vi "FPGAPowerMeasurement4.vi"() -> ()   [LabVIEW 2009]
uses:
  <vilib>/Waveform/DWDTOps.llb/Digital Pattern Generator (Toggle).vi
  <vilib>/express/express analysis/Spectral/XNode/ExpressSpectralMeasurementsBlockNode.xnode
  <vilib>/express/express analysis/Spectral/Block/exnSpectralBlock spectral measurements peak poly.vi
  <vilib>/express/express analysis/Spectral/Block/exnSpectralBlock spectral measurements peak DDT.vi
panel:
  out "Waveform Graph 2":dynamicdata(graph)
  out "Waveform Graph":dynamicdata(graph)
  out "Average Voltage":dbl
  out "Voltage At Power":dynamicdata(graph)
  out "Voltage at FPGA":dynamicdata(graph)
  out "Power":dynamicdata(graph)
  out "Average Power":dbl
  out "Average Voltage":dbl
  out "Average Current":dbl
  out "Current":dynamicdata(graph)
  in  "stop":bool
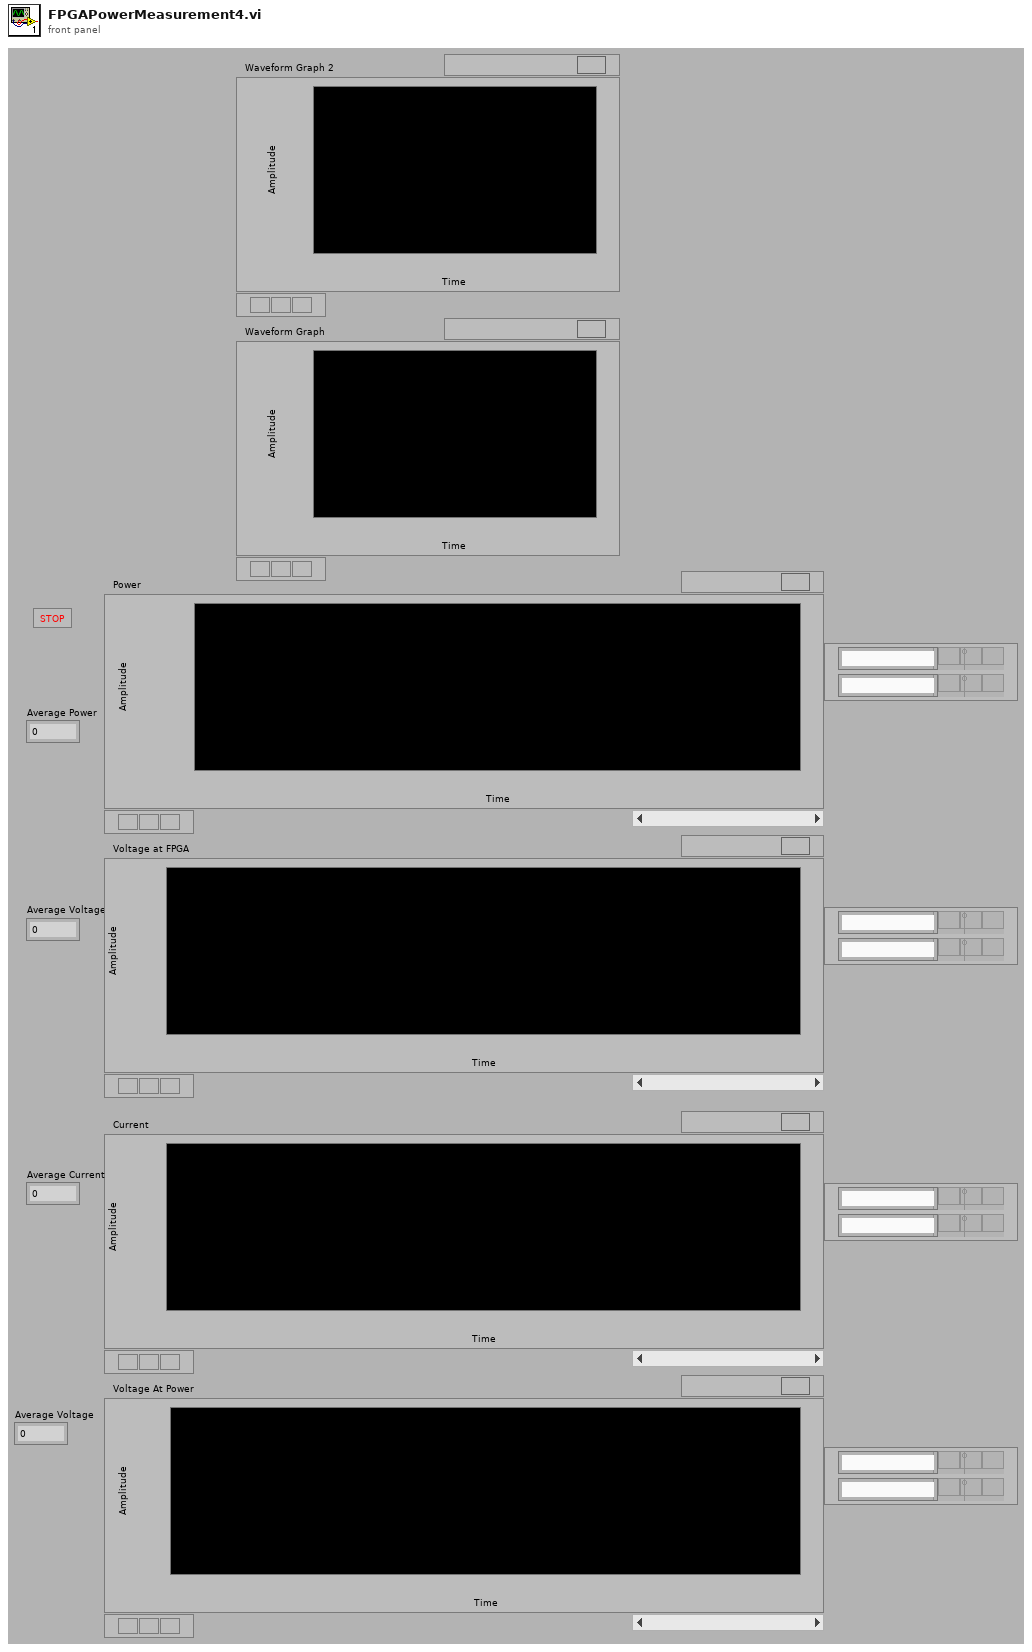
[diagram p1: front panel]
types:
  T1 = typedef "LVTextColorsTypeDef.ctl" = cluster{"Text Color":u32, "Background Color":u32}
  T2 = typedef "LVRangeTypeDef.ctl" = cluster{"Minimum":dbl, "Maximum":dbl, "Increment":dbl, "Minor Increment":dbl, "Start":dbl}
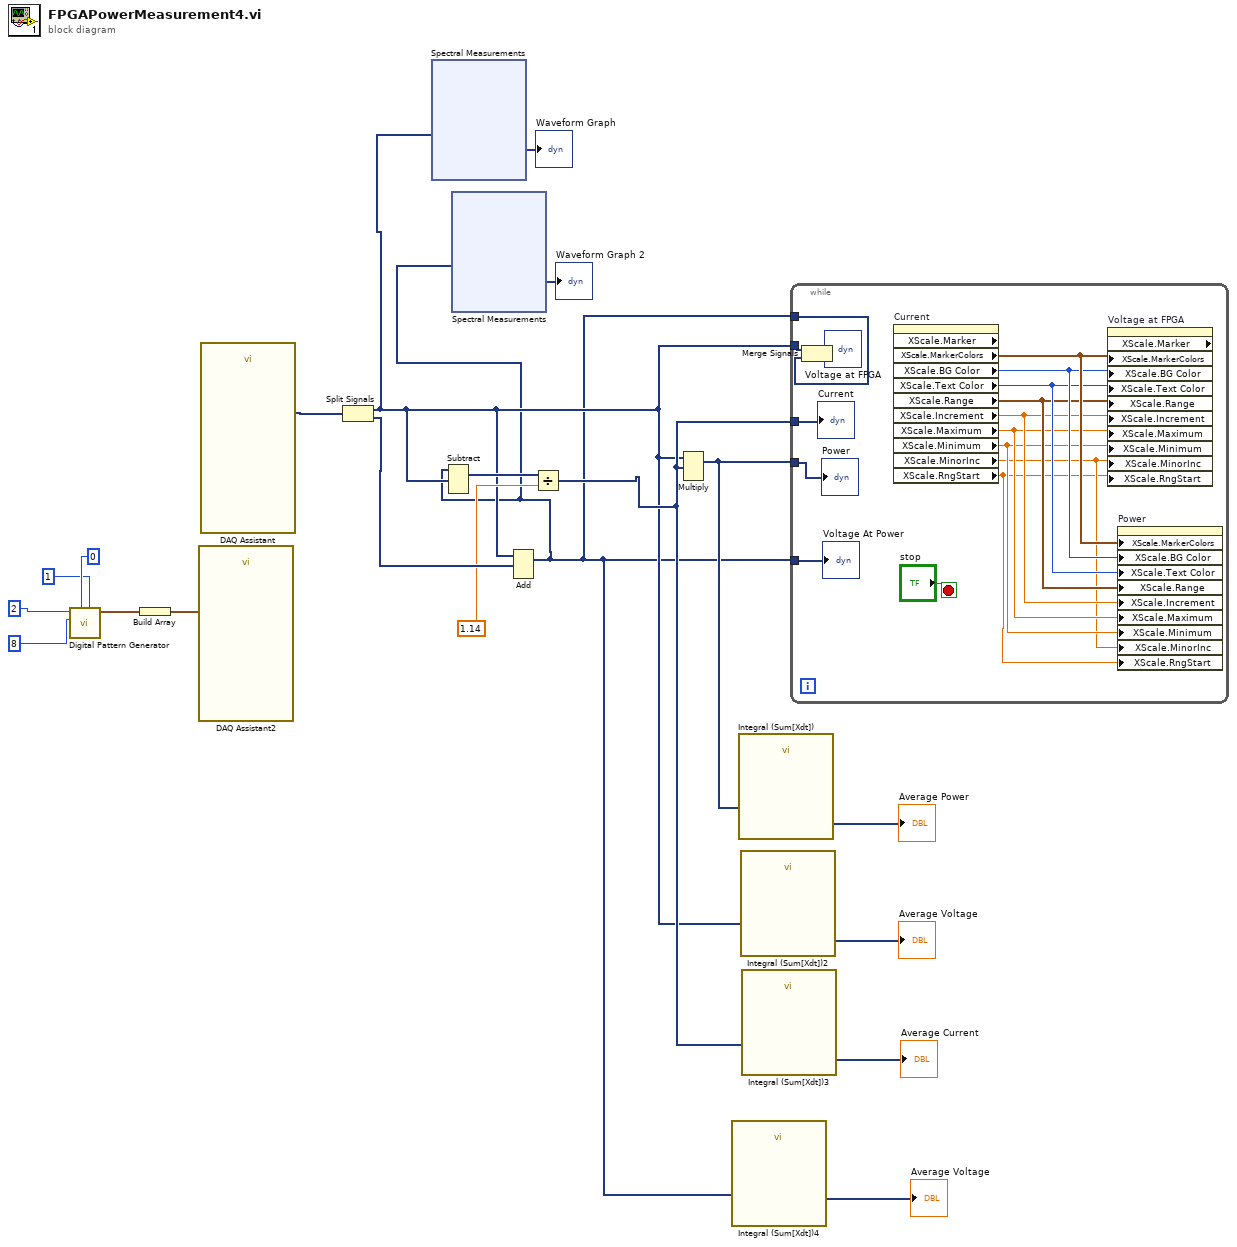
[diagram p0: block diagram]
diagram:
  n1 = call-poly <vilib>:"Digital Pattern Generator.vi"("value 2"=1, "value 1"=0, "number of signals"=8, "number of samples"=2) -> ("digital waveform"=w14:digitalwaveform)  [unwired: 6 in, 1 out]
  n2 = Build Array(w14) -> (w15:digitalwaveform[])
  n3 = call "DAQ Assistant2"("data"=w15) -> ()  [unwired: 17 in, 2 out]
  n4 = call "DAQ Assistant"() -> ("data"=w16:dynamicdata)  [unwired: 17 in, 2 out]
  n5 = Split Signals(w16) -> (w2:dynamicdata, w9:dynamicdata)  [unwired: 2 in]
  n6 = xnode "Spectral Measurements"("Signals"=w2) -> ("FFT - (Peak)"=→"Waveform Graph":dynamicdata)  [unwired: 1 in, 2 out]
  n7 = Add(1:w9, 2:w2) -> (0:w1:dynamicdata)  [unwired: 1 in, 1 out]
  n8 = Subtract(1:w2, 2:w1) -> (0:w7:dynamicdata)  [unwired: 1 in, 1 out]
  n9 = xnode "Spectral Measurements"("Signals"=w1) -> ("FFT - (Peak)"=→"Waveform Graph 2":dynamicdata)  [unwired: 1 in, 2 out]
  n10 = Divide(x=w7, y=1.14) -> (x/y=w5:dynamicdata)
  n11 = Multiply(1:w5, 2:w2) -> (0:w20:dynamicdata)  [unwired: 1 in, 1 out]
  n12 = call "Integral (Sum[Xdt])4"("Signals"=w1) -> ("Result"=→"Average Voltage":dynamicdata)  [unwired: 5 in, 1 out]
  n13 = call "Integral (Sum[Xdt])"("Signals"=w20) -> ("Result"=→"Average Power":dynamicdata)  [unwired: 5 in, 1 out]
  n14 = call "Integral (Sum[Xdt])2"("Signals"=w2) -> ("Result"=→"Average Voltage":dynamicdata)  [unwired: 5 in, 1 out]
  n15 = call "Integral (Sum[Xdt])3"("Signals"=w5) -> ("Result"=→"Average Current":dynamicdata)  [unwired: 5 in, 1 out]
  n16 = while {
    tunnel: w2 -> [w34]
    tunnel: w5 -> [w35]
    tunnel: w20 -> [w33]
    tunnel: w1 -> [w23]
    tunnel: w1 -> [w21]
    stop <- "stop" stop-if-true
    n17 = Merge Signals(w34, w21) -> (→"Voltage at FPGA":dynamicdata)
    n18 = property on="Current" class="WFGraph (strict)" props=["XScale", "Marker", "XScale", "MarkerColors", "XScale", "BG Color", "XScale", "Text Color", "XScale", "Range", "XScale", "Increment", "XScale", "Maximum", "XScale", "Minimum", "XScale", "MinorInc", "XScale", "RngStart"]() -> ("XScale.MarkerColors"=w32:T1, "XScale.BG Color"=w31:u32, "XScale.Text Color"=w30:u32, "XScale.Range"=w29:T2, "XScale.Increment"=w28:dbl, "XScale.Maximum"=w27:dbl, "XScale.Minimum"=w26:dbl, "XScale.MinorInc"=w25:dbl, "XScale.RngStart"=w24:dbl)  [unwired: 2 in, 3 out]
    n19 = property on="Voltage at FPGA" class="WFGraph (strict)" props=["XScale", "Marker", "XScale", "MarkerColors", "XScale", "BG Color", "XScale", "Text Color", "XScale", "Range", "XScale", "Increment", "XScale", "Maximum", "XScale", "Minimum", "XScale", "MinorInc", "XScale", "RngStart"]("XScale.MarkerColors"=w32, "XScale.BG Color"=w31, "XScale.Text Color"=w30, "XScale.Range"=w29, "XScale.Increment"=w28, "XScale.Maximum"=w27, "XScale.Minimum"=w26, "XScale.MinorInc"=w25, "XScale.RngStart"=w24) -> ()  [unwired: 2 in, 3 out]
    n20 = property on="Power" class="WFGraph (strict)"("XScale.MarkerColors"=w32, "XScale.BG Color"=w31, "XScale.Text Color"=w30, "XScale.Range"=w29, "XScale.Increment"=w28, "XScale.Maximum"=w27, "XScale.Minimum"=w26, "XScale.MinorInc"=w25, "XScale.RngStart"=w24) -> ()  [unwired: 2 in, 2 out]
    "Current" <- w35
    "Power" <- w33
    "Voltage At Power" <- w23
  }
